vi "AnÇmomätre.vi"(9 "vents":dbl) -> (1 "Vitesse (en m/s)":dbl, 2 "Nombre impulsion":dbl)   [LabVIEW 2017]
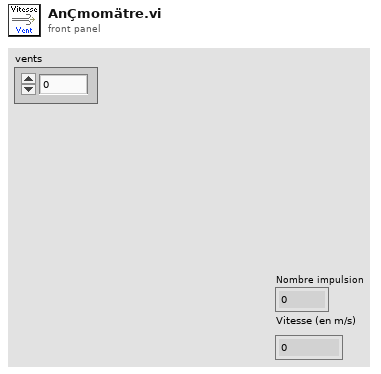
[diagram p1: front panel]
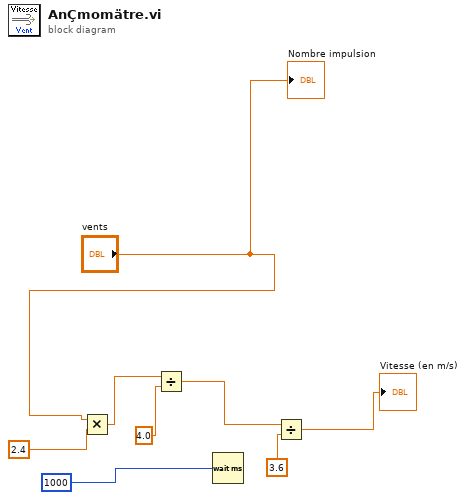
[diagram p0: block diagram]
diagram:
  n1 = Multiply(x="vents", y=2.4) -> (x*y=w5:dbl)
  n2 = Divide(x=w5, y=4.0) -> (x/y=w3:dbl)
  n3 = Wait (ms)(milliseconds to wait=u32 1000 ("attente (ms)")) -> ()  [unwired: 1 out]
  n4 = Divide(x=w3, y=3.6) -> (x/y=→"Vitesse (en m/s)":dbl)
  "Nombre impulsion" <- "vents"
